vi "ET2604 - Read From Register Floating Point.vi"(7 "Num Of Reg (1)":u16=1 min=1 step=1, 8 "error in (no error)":errorcluster, 9 "Register Address (0)":u16, 10 "Unit Address (1)":u8=1, 11 "VISA session":refnum<visa-resource-name>) -> (0 "error out":errorcluster, 2 "Data":sgl[](array[numeric]) format="%.3f", 3 "dup VISA session":refnum<visa-resource-name>)   [LabVIEW 2017]
doc: "This VI reads value from specified registers of specified unit."
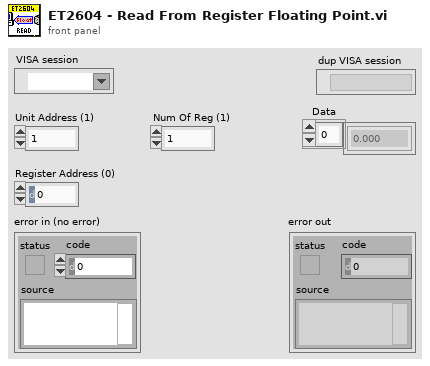
[diagram p1: front panel]
types:
  T1 = enum16{"By The Number of Bytes", "Copy Of the Sent Message"}
  T2 = cluster{"Read Buffer[0]":u8, "Read Buffer[1]":u8}
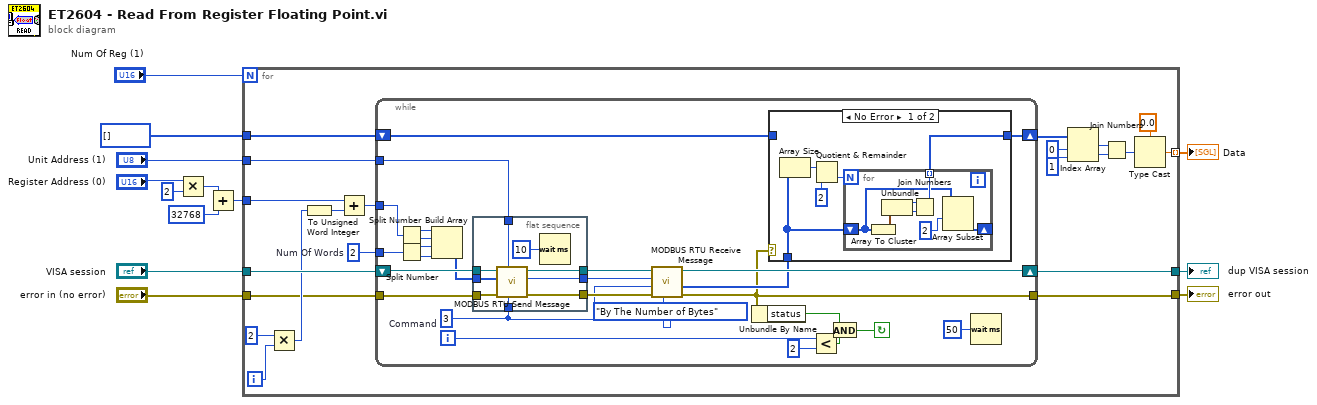
[diagram p0: block diagram]
diagram:
  n1 = Multiply(x="Register Address (0)", y=u16 2) -> (x*y=w6:u16)
  n2 = Add(x=w6, y=u16 32768) -> (x+y=w1:u16)
  n3 = for {
    N: "Num Of Reg (1)" -> [_]
    tunnel: "VISA session" -> [w34]
    tunnel: [w33] -> w12
    tunnel: u16[] [] -> [w32]
    tunnel: "error in (no error)" -> [w15]
    tunnel: [w14] -> w9
    tunnel: "Unit Address (1)" -> [w31]
    tunnel: w1 -> [w21]
    tunnel: [w23] -> w2 mode=indexing
    i -> [w20]
    w30 = u16 2  # Num Of Words
    n4 = Multiply(x=2, y=w20) -> (x*y=w18:i32)
    n5 = To Unsigned Word Integer(number=w18) -> (unsigned 16bit integer=w17:u16)
    n6 = Add(x=w21, y=w17) -> (x+y=w22:u16)
    n7 = while {
      tunnel: w31 -> [w46]
      shift-right: [w41] -> w33
      shift-left: w34 -> [w60]
      tunnel: w30 -> [w49]
      shift-right: [w51] -> w16
      shift-left: w32 -> [w50]
      tunnel: w22 -> [w44]
      tunnel: w15 -> [w43]
      tunnel: [w39] -> w14
      i -> [w57]
      stop <- w58 continue-if-true
      w37 = u8 3  # Command
      n8 = Split Number(x=w44) -> (hi(x)=w53:u8, lo(x)=w52:u8)
      n9 = Split Number(x=w49) -> (hi(x)=w48:u8, lo(x)=w47:u8)
      n10 = Build Array(w53, w52, w48, w47) -> (w54:u8[])
      n11 = flat-sequence {
        tunnel: [w64] -> w38
        tunnel: [w67] -> w42
        tunnel: w60 -> [w66]
        tunnel: w54 -> [w62]
        tunnel: w46 -> [w68]
        tunnel: [w65] -> w36
        tunnel: w43 -> [w63]
        tunnel: w37 -> [w61]
        frame #0 {
          n12 = call "MODBUS RTU Send Message.vi"("Command (0)"=w61, "Unit Address (1)"=w68, "error in (no error)"=w63, "Message (empty array)"=w62, "VISA session"=w66) -> ("error out"=w64:errorcluster, "Length Of Sent MSG"=w65:u8, "dup VISA session"=w67:refnum<visa-resource-name>)  [unwired: 4 in]
          n13 = Wait (ms)(milliseconds to wait=u32 10) -> ()  [unwired: 1 out]
        }
      }
      n14 = call "MODBUS RTU Receive Message.vi"("Receive Message Type (0: By The Number Of Bytes)"=T1."By The Number of Bytes" ("Receive Message Type"), "error in (no error)"=w38, "Sent Command (0)"=w37, "Length Of Sent MSG (0)"=w36, "VISA session"=w42) -> ("error out"=w39:errorcluster, "Read Buffer"=w40:u8[], "dup VISA session"=w41:refnum<visa-resource-name>)  [unwired: 4 in]
      n15 = Unbundle By Name(w39) -> ("status"=w59:bool)
      n16 = case shown="No Error" w39 {
        tunnel: w40 -> [w74 _]
        tunnel: [w73 w82] -> w51
        tunnel: w50 -> [_ w82]
        frame No Error {
          n17 = Array Size(array=w74) -> (size(s)=w72:i32)
          n18 = Quotient & Remainder(x=w72, y=2) -> (floor(x/y)=w70:i32)  [unwired: 1 out]
          n19 = for {
            N: w70 -> [_]
            shift-right: [w76] -> _
            shift-left: w74 -> [w77]
            tunnel: [w78] -> w73 mode=indexing
            n20 = Array To Cluster(array=w77) -> (cluster=w81:T2)
            n21 = Unbundle(w81) -> ("Read Buffer[0]"=w79:u8, "Read Buffer[1]"=w80:u8)
            n22 = Join Numbers(hi=w79, lo=w80) -> ((hi.lo)=w78:u16)
            n23 = Array Subset(array=w77, index=2) -> (w76:u8[])  [unwired: 1 in]
          }
        }
        frame Error {
        }
      }
      n24 = Less?(x=w57, y=2) -> (x < y?=w56:bool)
      n25 = And(x=w59, y=w56) -> (x .and. y?=w58:bool)
      n26 = Wait (ms)(milliseconds to wait=u32 50) -> ()  [unwired: 1 out]
    }
    n27 = Index Array(array=w16, index #1=0 ("index"), index #2=1 ("index")) -> (element #1=w28:u16, element #2=w29:u16)
    n28 = Join Numbers(hi=w28, lo=w29) -> ((hi.lo)=w24:u32)
    n29 = Type Cast(type=sgl 0.0, x=w24) -> (*(type *) &x=w23:sgl)
  }
  "error out" <- w9
  "dup VISA session" <- w12
  "Data" <- w2
